vi "Set value and frequnecy AR.vi"(6 "Voltage frequnecy limit (none)":T1(ring), 7 "Ignore intr. errors (false)":bool, 8 "error in":errorcluster, 9 "Frequency [Hz]":dbl=10.0 min=10.0 max=1000000.0, 10 "Value":dbl, 11 "VISA resource name":refnum<visa-resource-name>) -> (0 "error out":errorcluster, 2 "Setup failed":bool, 3 "VISA resource name out":refnum<visa-resource-name>)   [LabVIEW 2020, in "Datron D4xxx.lvlib"]
doc: "Sets value using \"Set value AR\" VI and then desired frequency using \"Set frequency\". Options are same as in theese VIs."
uses:
  Datron D4xxx.lvlib
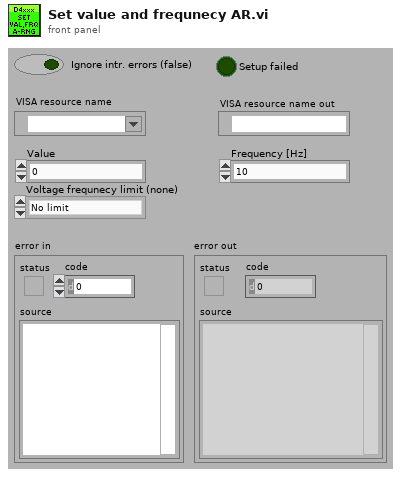
[diagram p1: front panel]
types:
  T1 = enum16{"No limit", "Always to 1kHz", "D4800", "D4805", "D4808"}
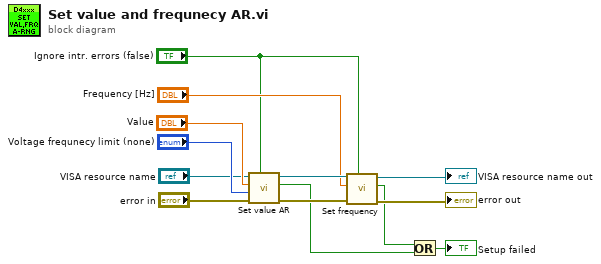
[diagram p0: block diagram]
diagram:
  n1 = call "Set value AR.vi"("Ignore range overflow error (false)"="Ignore intr. errors (false)", "error in"="error in", "Voltage frequnecy limit (none)"="Voltage frequnecy limit (none)", "Value"="Value", "VISA resource name"="VISA resource name") -> ("error out"=w11:errorcluster, "Set value failed"=w1:bool, "VISA resource name out"=w10:refnum<visa-resource-name>)  [unwired: 4 in]
  n2 = call "Set frequency.vi"("Ignore out of range error (false)"="Ignore intr. errors (false)", "error in"=w11, "Frequency"="Frequency [Hz]", "VISA resource name"=w10) -> ("error out"=→"error out":errorcluster, "Set frequency failed"=w2:bool, "VISA resource name out"=→"VISA resource name out":refnum<visa-resource-name>)  [unwired: 5 in]
  n3 = Or(x=w2, y=w1) -> (x .or. y?=→"Setup failed":bool)
